vi "CreatePacket.vi"(8 "error in":errorcluster, 10 "data":u8[](array[numeric]) format="%x", 11 "command":u8) -> (0 "error out":errorcluster, 2 "output cluster":T1 {"buffer" format="%x"}, 3 "Command String":string)   [LabVIEW 2019]
panel:
  out "Comman Bytes":u8[](array[numeric])
  in  "CommandPacket":T1 {"buffer" format="%x"}
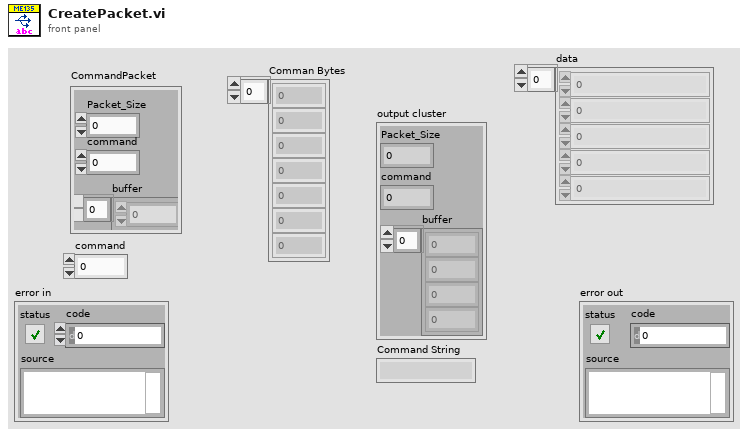
[diagram p1: front panel]
types:
  T1 = cluster{"Packet_Size":u8, "command":u8, "buffer":u8[]}
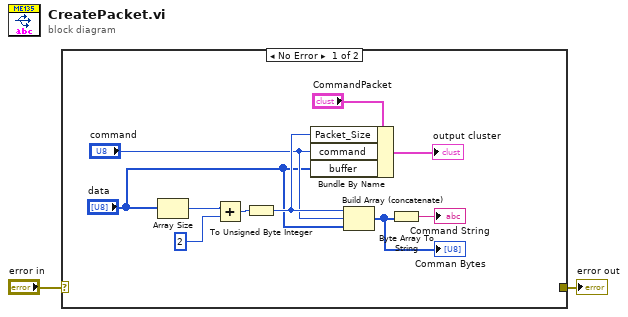
[diagram p0: block diagram]
diagram:
  n1 = case shown="No Error" "error in" {
    selector: "error in" -> [_ w13]
    tunnel: [_ w13] -> w1
    frame No Error {
      n2 = Array Size(array="data") -> (size(s)=w11:i32)
      n3 = Add(x=w11, y=2) -> (x+y=w9:i32)
      n4 = To Unsigned Byte Integer(number=w9) -> (unsigned 8bit integer=w7:u8)
      n5 = Bundle By Name(cluster="CommandPacket", "Packet_Size"=w7, "command"="command", "buffer"="data") -> (→"output cluster":T1)
      n6 = Build Array (concatenate)(w7, "command", "data") -> (w3:u8[])
      "Comman Bytes" <- w3
      n7 = Byte Array To String(unsigned byte array=w3) -> (string=→"Command String":string)
    }
    frame Error {
    }
  }
  "error out" <- w1
